vi "CurrentVI_FGV.vi"(7 "Mode":enum16{"Get", "Set"}(ring), 8 "error in (no error)":errorcluster, 11 "VI in":refnum<vi>) -> (0 "error out":errorcluster, 3 "VI out":refnum<vi>)   [LabVIEW 2021]
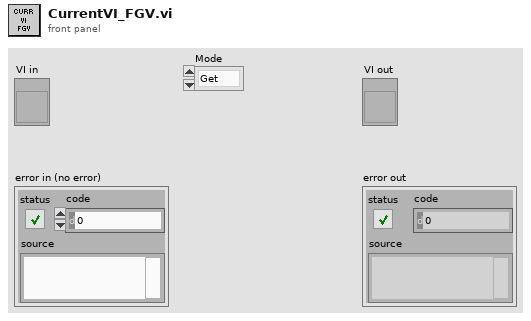
[diagram p1: front panel]
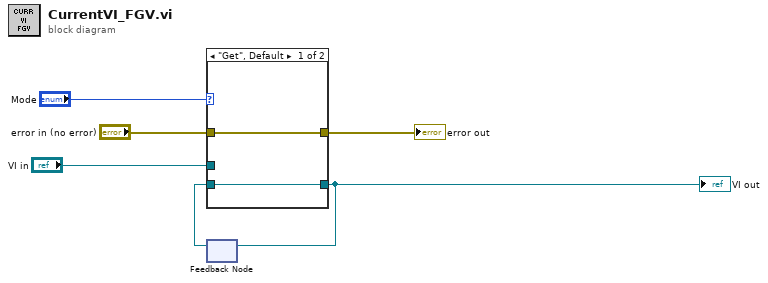
[diagram p0: block diagram]
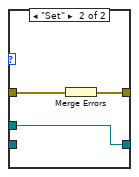
[diagram p2: hidden frame]
diagram:
  n1 = feedback #1() -> (w2:refnum<vi>)  [unwired: 1 in]
  n2 = case shown="\"Get\", Default" "Mode" {
    tunnel: "error in (no error)" -> [w8 w11]
    tunnel: [w8 w10] -> w4
    tunnel: "VI in" -> [_ w9]
    tunnel: [w7 w9] -> w1
    tunnel: w2 -> [w7 _]
    frame "Get", Default {
    }
    frame "Set" {
      n3 = Merge Errors(w11) -> (w10:errorcluster)
    }
  }
  "VI out" <- w1
  "error out" <- w4
  n4 = feedback-in #1(w1) -> ()
